vi "Static Write.vi"(8 "error in (no error)":errorcluster, 10 "Value":sgl, 11 "Abs_Single Float in":refnum<class "Abs_Single Float.lvclass">) -> (0 "error out":errorcluster, 3 "Abs_Single Float out":refnum<class "Abs_Single Float.lvclass">)   [LabVIEW 2021, in "Abs_Single Float.lvclass"]
uses:
  Abs_Single Float.lvclass
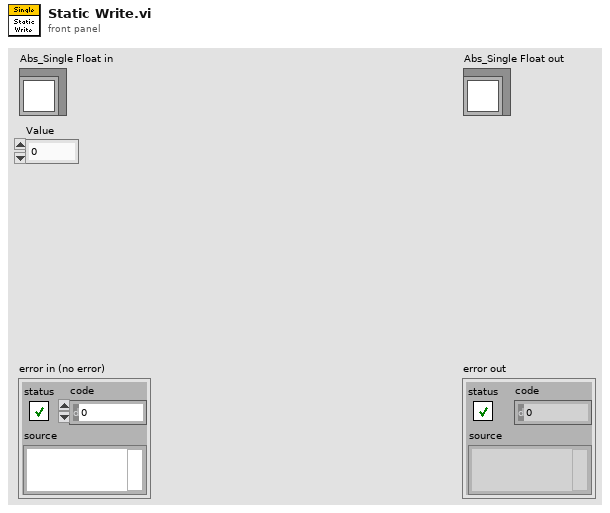
[diagram p1: front panel]
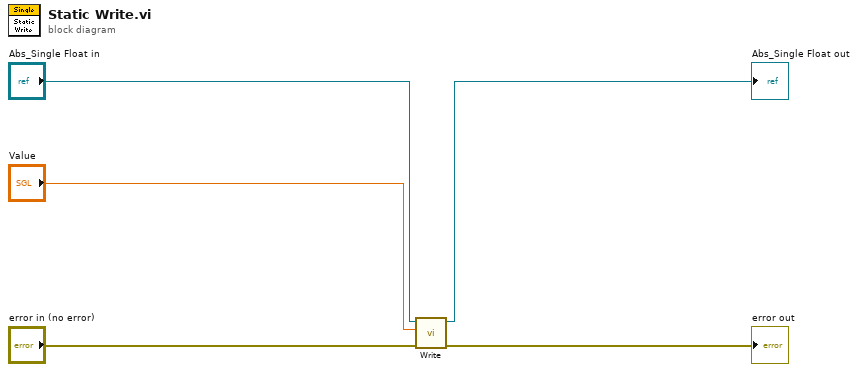
[diagram p0: block diagram]
diagram:
  n1 = call-dynamic "Write.vi"("error in (no error)"="error in (no error)", "Value"="Value", "Double Float.lvclass_340760 in"="Abs_Single Float in") -> ("error out"=→"error out":errorcluster, "Double Float.lvclass_340760 out"=→"Abs_Single Float out":refnum<class "Abs_Single Float.lvclass">)  [unwired: 7 in]
